vi "Build One Term Compare Types.vi"(11 "Comparison Name":string) -> ()   [LabVIEW 2019]
uses:
  <vilib>/numeric/LVNumericRepresentation.ctl
  71b9e51f-dfc8-458f-9837-ddab78837e89.vi
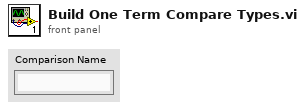
[diagram p1: front panel]
types:
  T1 = typedef "LVNumericRepresentation.ctl" = enum32{"Extended Precision", "Double Precision", "Single Precision", "Long", "Word", "Byte", "Unsigned Long", "Unsigned Word", "Unsigned Byte", "Complex Extended", "Complex Double", "Complex Single", "Quad", "Unsigned Quad", "Fixed-Point"}
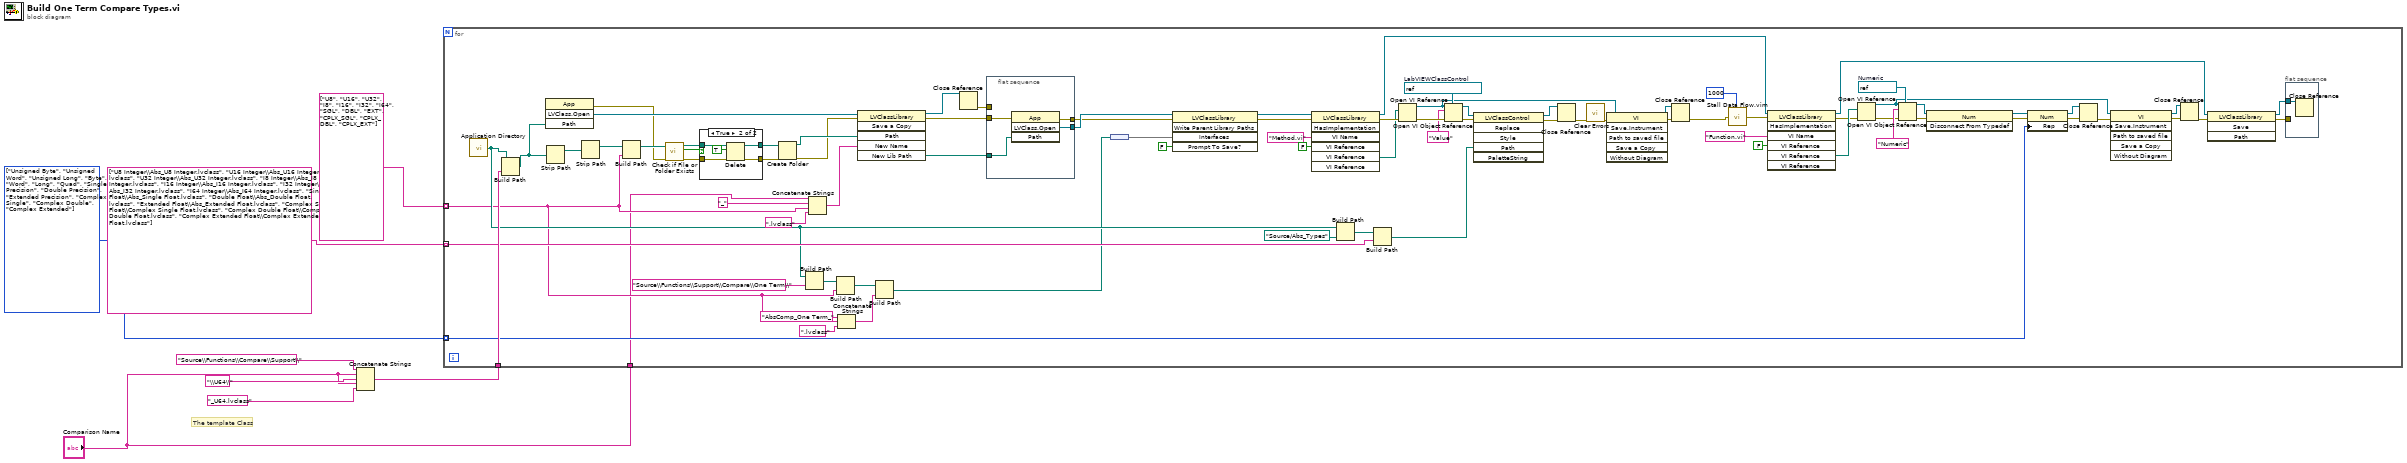
[diagram p0: block diagram]
diagram:
  w6 = T1[] [enum."Unsigned Byte", enum."Unsigned Word", enum."Unsigned Long", enum."Byte", enum."Word", enum."Long", enum."Quad", enum."Single Precision", enum."Double Precision", enum."Extended Precision", enum."Complex Single", enum."Complex Double", enum."Complex Extended"] items=["Extended Precision", "Double Precision", "Single Precision", "Long", "Word", "Byte", "Unsigned Long", "Unsigned Word", "Unsigned Byte", "Complex Extended", "Complex Double", "Complex Single", "Quad", "Unsigned Quad", "Fixed-Point"] ("Representation")
  # "The template Class"
  n1 = Concatenate Strings("Source\\Functions\\Compare\\Support\\", "Comparison Name", "\\U64\\", "Comparison Name", "_U64.lvclass") -> (w2:string)
  n2 = for {
    tunnel: string[] ["U8", "U16", "U32", "I8", "I16", "I32", "I64", "SGL", "DBL", "EXT", "CPLX_SGL", "CPLX_DBL", "CPLX_EXT"] -> [w27] mode=indexing
    tunnel: w2 -> [w72]
    tunnel: string[] ["U8 Integer\\Abs_U8 Integer.lvclass", "U16 Integer\\Abs_U16 Integer.lvclass", "U32 Integer\\Abs_U32 Integer.lvclass", "I8 Integer\\Abs_I8 Integer.lvclass", "I16 Integer\\Abs_I16 Integer.lvclass", "I32 Integer\\Abs_I32 Integer.lvclass", "I64 Integer\\Abs_I64 Integer.lvclass", "Single Float\\Abs_Single Float.lvclass", "Double Float\\Abs_Double Float.lvclass", "Extended Float\\Abs_Extended Float.lvclass", "Complex Single Float\\Complex Single Float.lvclass", "Complex Double Float\\Complex Double Float.lvclass", "Complex Extended Float\\Complex Extended Float.lvclass"] -> [w64] mode=indexing
    tunnel: w6 -> [w48] mode=indexing
    tunnel: "Comparison Name" -> [w9]
    w49 = refnum<vi> refnum  # Numeric
    w58 = refnum<vi> refnum  # LabVIEWClassControl
    n3 = call <vilib>:"Application Directory.vi"() -> ("Application Directory"=w31:path)
    n4 = Build Path(base path=w31, name or relative path=w72) -> (appended path=w73:path)
    n5 = invoke class="App" method="LVClass.Open"("Path"=w73) -> (error out=w78:errorcluster, "LVClass.Open"=w91:refnum<vi>)  [unwired: 3 in, 2 out]
    n6 = Strip Path(path=w73) -> (stripped path=w89:path)  [unwired: 1 out]
    n7 = Strip Path(path=w89) -> (stripped path=w88:path)  [unwired: 1 out]
    n8 = Build Path(base path=w88, name or relative path=w27) -> (appended path=w84:path)
    n9 = call <vilib>:"Check if File or Folder Exists.vi"("error in (no error)"=w78, "path"=w84) -> ("error out"=w77:errorcluster, "file or folder exists?"=w86:bool, "dup path"=w87:path)  [unwired: 7 in]
    n10 = case shown="True" w86 {
      tunnel: w87 -> [w98 w103]
      tunnel: [w98 w101] -> w85
      tunnel: w77 -> [w97 w100]
      tunnel: [w97 w99] -> w76
      frame False {
      }
      frame True {
        n11 = Delete(path (use dialog)=w103, entire hierarchy (F)=TRUE, error in=w100) -> (deleted path=w101:path, error out=w99:errorcluster)  [unwired: 2 in, 1 out]
      }
    }
    n12 = Create Folder(path (use dialog)=w85, error in=w76) -> (created path=w83:path, error out=w75:errorcluster)  [unwired: 1 in, 1 out]
    n13 = Build Path(base path=w31, name or relative path="Source\\Functions\\Support\\Compare\\One Term\\") -> (appended path=w30:path)
    n14 = Concatenate Strings(w9, "_", w27, ".lvclass") -> (w71:string)
    n15 = Build Path(base path=w30, name or relative path=w27) -> (appended path=w29:path)
    n16 = Concatenate Strings("AbsComp_One Term_" ("string"), w27, ".lvclass") -> (w25:string)
    n17 = invoke class="LVClassLibrary" method="Save a Copy"(reference=w91, error in=w75, "Path"=w83, "New Name"=w71) -> (reference out=w90:refnum<vi>, error out=w79:errorcluster, "New Lib Path"=w80:path)  [unwired: 2 in, 3 out]
    n18 = Build Path(base path=w29, name or relative path=w25) -> (appended path=w23:path)
    n19 = Close Reference(reference=w90) -> (error out=w74:errorcluster)  [unwired: 1 in]
    n20 = flat-sequence {
      tunnel: w80 -> [w95]
      tunnel: w79 -> [w96]
      tunnel: w74 -> [_]
      tunnel: [w93] -> w40
      tunnel: [w94] -> w24
      frame #0 {
        n21 = invoke class="App" method="LVClass.Open"(error in=w96, "Path"=w95) -> (error out=w94:errorcluster, "LVClass.Open"=w93:refnum<vi>)  [unwired: 2 in, 2 out]
      }
    }
    n22 = node(w23) -> (w22:set{path})
    n23 = invoke class="LVClassLibrary" method="Write Parent Library Paths"(reference=w40, error in=w24, "Interfaces"=w22, "Prompt To Save?"=FALSE) -> (reference out=w39:refnum<vi>, error out=w38:errorcluster)  [unwired: 1 in, 3 out]
    n24 = invoke class="LVClassLibrary" method="HasImplementation"(reference=w39, error in=w38, "VI Name"="Method.vi", "VI Reference"=FALSE ("Consider Parents?")) -> (reference out=w42:refnum<vi>, error out=w69:errorcluster, "VI Reference"=w68:path)  [unwired: 3 in, 4 out]
    n25 = Build Path(base path=w31, name or relative path=path "Source/Abs_Types") -> (appended path=w65:path)
    n26 = Build Path(base path=w65, name or relative path=w64) -> (appended path=w41:path)
    n27 = Open VI Reference(vi path=w68, error in (no error)=w69) -> (vi reference=w15:refnum<vi>, error out=w63:errorcluster)  [unwired: 4 in]
    n28 = Open VI Object Reference(7:w58, 8:w63, 10:"Value" ("name/order"), 11:w15) -> (0:w61:errorcluster, 3:w60:refnum<vi>)
    n29 = invoke class="LVClassControl" method="Replace"(reference=w60, error in=w61, "Path"=w41) -> (reference out=w59:refnum<vi>, error out=w57:errorcluster)  [unwired: 3 in, 4 out]
    n30 = Close Reference(reference=w59, error in (no error)=w57) -> (error out=w56:errorcluster)
    n31 = call <vilib>:"Clear Errors.vi"("error in (no error)"=w56) -> ("error out"=w16:errorcluster)  [unwired: 5 in, 1 out]
    n32 = invoke class="VI" method="Save.Instrument"(reference=w15, error in=w16) -> (reference out=w14:refnum<vi>, error out=w17:errorcluster)  [unwired: 4 in, 4 out]
    n33 = Close Reference(reference=w14, error in (no error)=w17) -> (error out=w45:errorcluster)
    n34 = call "Stall Data Flow.vim"("value in"=w45, "milliseconds to wait"=u32 1000) -> ("value out"=w44:errorcluster)  [unwired: 1 out]
    n35 = invoke class="LVClassLibrary" method="HasImplementation"(reference=w42, error in=w44, "VI Name"="Function.vi", "VI Reference"=FALSE ("Consider Parents?")) -> (reference out=w34:refnum<vi>, error out=w52:errorcluster, "VI Reference"=w53:path)  [unwired: 3 in, 4 out]
    n36 = Open VI Reference(vi path=w53, error in (no error)=w52) -> (vi reference=w10:refnum<vi>, error out=w50:errorcluster)  [unwired: 4 in]
    n37 = Open VI Object Reference(7:w49, 8:w50, 10:"Numeric" ("name/order"), 11:w10) -> (0:w18:errorcluster, 3:w19:refnum<vi>)
    n38 = invoke class="Num" method="Disconnect From Typedef"(reference=w19, error in=w18) -> (reference out=w21:refnum<vi>, error out=w20:errorcluster)  [unwired: 1 in, 1 out]
    n39 = property class="Num"(reference=w21, error in=w20, "Rep"=w48) -> (reference out=w46:refnum<vi>, error out=w47:errorcluster)
    n40 = Close Reference(reference=w46, error in (no error)=w47) -> (error out=w11:errorcluster)
    n41 = invoke class="VI" method="Save.Instrument"(reference=w10, error in=w11) -> (reference out=w13:refnum<vi>, error out=w12:errorcluster)  [unwired: 4 in, 4 out]
    n42 = Close Reference(reference=w13, error in (no error)=w12) -> (error out=w36:errorcluster)
    n43 = invoke class="LVClassLibrary" method="Save"(reference=w34, error in=w36) -> (reference out=w33:refnum<vi>, error out=w35:errorcluster)  [unwired: 2 in, 2 out]
    n44 = flat-sequence {
      tunnel: w33 -> [w92]
      tunnel: w35 -> [_]
      frame #0 {
        n45 = Close Reference(reference=w92) -> ()  [unwired: 1 in, 1 out]
      }
    }
  }
